vi "GetRobotPose.vi"() -> ()   [LabVIEW 2019]
uses:
  refnums.vi
  GRNF_GenericMotor.vi
  dsinstructions.vi
  sensors.vi
  dsdata.vi
  autoinfo.vi
panel:
  out "Y Position (in)":dbl=94.7
  out "X Position (in)":dbl=509.2
  out "Robot Position":cluster{dbl[], dbl[]}(graph)
  out "Heading (deg)":dbl format="%#_13g"
  in  "Plot Data":bool
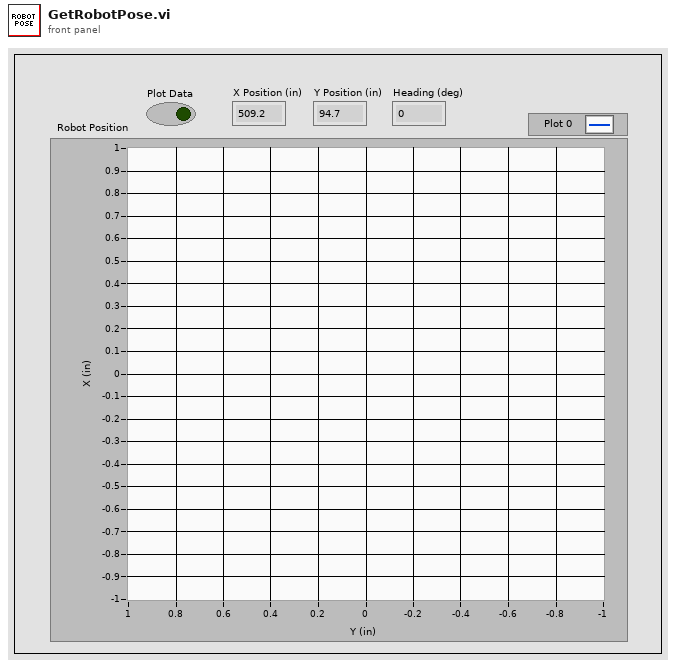
[diagram p1: front panel]
types:
  T1 = enum16{"Center", "North", "NorthWest", "West", "SouthWest", "South", "SouthEast", "East", "NorthEast"}
  T2 = typedef "WPI_MotorControlDeviceRef.ctl" = cluster{"DeviceStatus":errorcluster, "Type":T3, "PWM":cluster{"PWM Channel":T4, "DeadBand":T5}, "CAN":cluster{"Device Number":u8, "SetOutput VI Ref":variant, "GetOutput VI Ref":variant, "Enable VI Ref":variant, "Disable VI Ref":variant, "Data":variant}, "Invert":bool, "DIO PWM":cluster{"PWM \"Enable\" Channel":T4, "DIOChannel":T6, "PWM Rate":dbl}}
  T3 = typedef "WPI_MotorControlType.ctl" = enum16{"PWM", "CAN", "DIO PWM"}
  T4 = typedef "FPGA_DIOPWMChannel.ctl" = enum8{"PWM 0", "PWM 1", "PWM 2", "PWM 3", "PWM 4", "PWM 5", "PWM 6", "PWM 7", "PWM 8", "PWM 9", "PWM MXP 0", "PWM MXP 1", "PWM MXP 2", "PWM MXP 3", "PWM MXP 4", "PWM MXP 5", "PWM MXP 6", "PWM MXP 7", "PWM MXP 8", "PWM MXP 9", "Invalid"}
  T5 = typedef "WPI_PWMDeadband.ctl" = cluster{"Name":string, "maxPositivePwm":i32, "minPositivePwm":i32, "centerPwm":i32, "maxNegativePwm":i32, "minNegativePwm":i32, "angularRange":u16}
  T6 = typedef "FPGA_DIOChannel.ctl" = enum8{"DIO 0", "DIO 1", "DIO 2", "DIO 3", "DIO 4", "DIO 5", "DIO 6", "DIO 7", "DIO 8", "DIO 9", "DIO MXP 0", "DIO MXP 1", "DIO MXP 2", "DIO MXP 3", "DIO MXP 4", "DIO MXP 5", "DIO MXP 6", "DIO MXP 7", "DIO MXP 8", "DIO MXP 9", "DIO MXP 10", "DIO MXP 11", "DIO MXP 12", "DIO MXP 13", "DIO MXP 14", "DIO MXP 15", "SPI Port CS1", "SPI Port CS2", "SPI Port CS3", "SPI Port MISO", "SPI Port MOSI", "Invalid"}
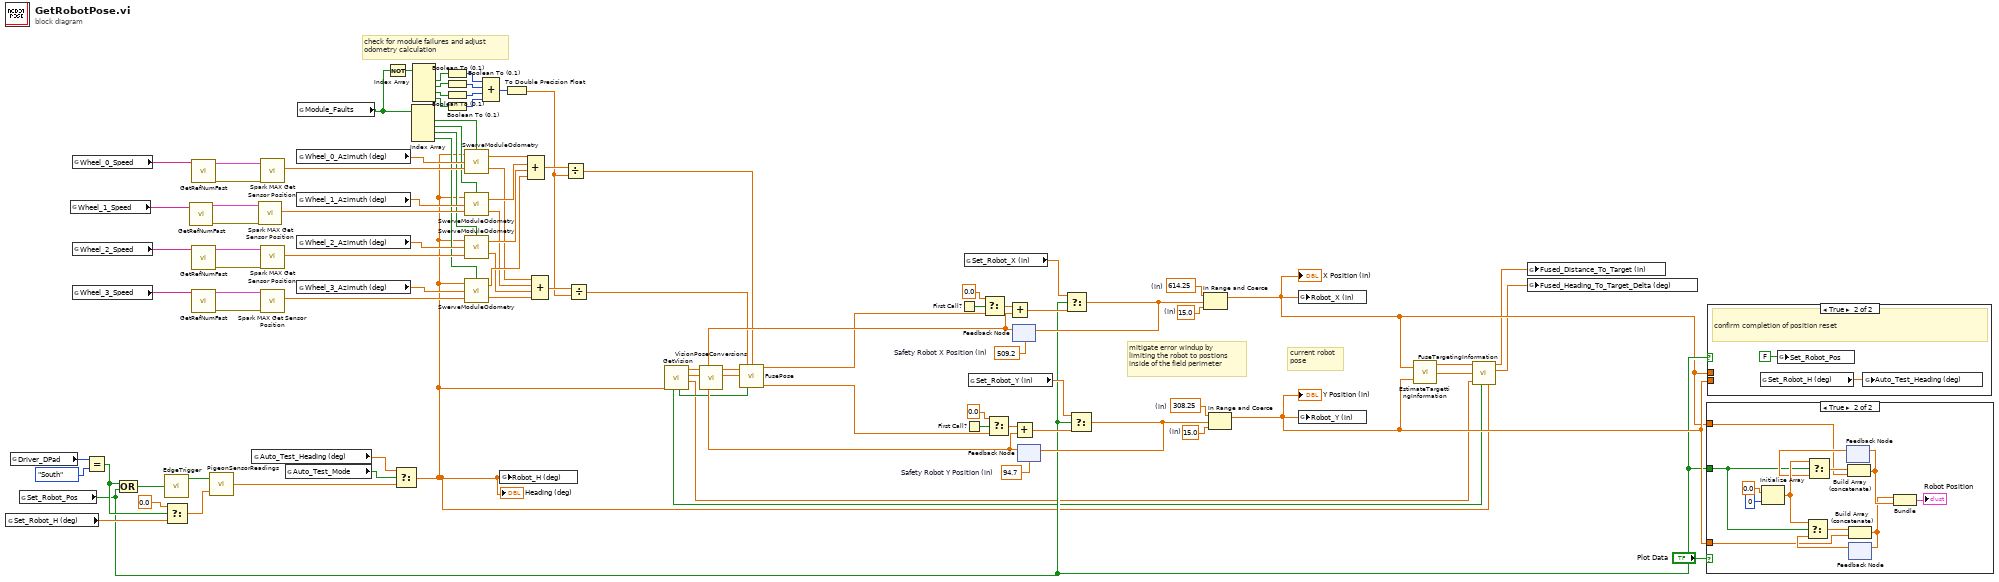
[diagram p0: block diagram]
diagram:
  w29 = 308.25  # (in)
  w30 = 15.0  # (in)
  w37 = 614.25  # (in)
  w38 = 15.0  # (in)
  w39 = 509.2  # Safety Robot X Position (in)
  w20 = 94.7  # Safety Robot Y Position (in)
  # "current robot\npose"
  # "mitigate error windup by\nlimiting the robot to postions\ninside of the field perimeter"
  # "check for module failures and adjust\nodometry calculation"
  n1 = global read "sensors.vi" "Set_Robot_H (deg)"() -> (w78:dbl)
  n2 = global read "dsinstructions.vi" "Driver_DPad"() -> (w54:T1)
  n3 = global read "sensors.vi" "Set_Robot_Pos"() -> (w12:bool)
  n4 = global read "refnums.vi" "Wheel_1_Speed"() -> (w46:string)
  n5 = global read "refnums.vi" "Wheel_0_Speed"() -> (w49:string)
  n6 = global read "refnums.vi" "Wheel_2_Speed"() -> (w43:string)
  n7 = global read "refnums.vi" "Wheel_3_Speed"() -> (w40:string)
  n8 = Equal?(x=w54, y=T1."South") -> (x = y?=w53:bool)
  n9 = Compound Arithmetic op=OR(w53, w12) -> (w77:bool)
  n10 = call "EdgeTrigger.vi"("Input Signal"=w77) -> ("Rising Edge Trigger"=w76:bool)  [unwired: 2 out]
  n11 = Select(t=0.0 ("f"), s=w53, f=w78) -> (s? t:f=w80:dbl)
  n12 = call-poly "GetRefNumFast.vi"("RefNum Name"=w46) -> ("Error"=w47:errorcluster, "Device Reference"=w48:T2)  [unwired: 5 in]
  n13 = call-poly "GetRefNumFast.vi"("RefNum Name"=w49) -> ("Error"=w50:errorcluster, "Device Reference"=w51:T2)  [unwired: 5 in]
  n14 = call-poly "GetRefNumFast.vi"("RefNum Name"=w43) -> ("Error"=w44:errorcluster, "Device Reference"=w45:T2)  [unwired: 5 in]
  n15 = call-poly "GetRefNumFast.vi"("RefNum Name"=w40) -> ("Error"=w41:errorcluster, "Device Reference"=w42:T2)  [unwired: 5 in]
  n16 = call "PigeonSensorReadings.vi"("Reset Yaw (deg)"=w80, "Reset Yaw"=w76) -> ("Yaw (deg)"=w57:dbl)
  n17 = global read "autoinfo.vi" "Auto_Test_Heading (deg)"() -> (w55:dbl)
  n18 = call <vilib>:"Spark MAX Get Sensor Position.vi"("error in (no error)"=w47, "MotorControlDevRef in"=w48) -> ("Sensor Position"=w94:dbl)  [unwired: 6 in, 3 out]
  n19 = call <vilib>:"Spark MAX Get Sensor Position.vi"("error in (no error)"=w50, "MotorControlDevRef in"=w51) -> ("Sensor Position"=w96:dbl)  [unwired: 6 in, 3 out]
  n20 = call <vilib>:"Spark MAX Get Sensor Position.vi"("error in (no error)"=w44, "MotorControlDevRef in"=w45) -> ("Sensor Position"=w93:dbl)  [unwired: 6 in, 3 out]
  n21 = call <vilib>:"Spark MAX Get Sensor Position.vi"("error in (no error)"=w41, "MotorControlDevRef in"=w42) -> ("Sensor Position"=w74:dbl)  [unwired: 6 in, 3 out]
  n22 = global read "dsdata.vi" "Auto_Test_Mode"() -> (w56:bool)
  n23 = global read "sensors.vi" "Wheel_0_Azimuth (deg)"() -> (w95:dbl)
  n24 = global read "sensors.vi" "Wheel_1_Azimuth (deg)"() -> (w92:dbl)
  n25 = global read "sensors.vi" "Wheel_2_Azimuth (deg)"() -> (w91:dbl)
  n26 = global read "sensors.vi" "Wheel_3_Azimuth (deg)"() -> (w75:dbl)
  n27 = global read "sensors.vi" "Module_Faults"() -> (w73:bool[])
  n28 = Not(x=w73) -> (.not. x?=w72:bool[])
  n29 = Select(t=w55, s=w56, f=w57) -> (s? t:f=w5:dbl)
  "Heading (deg)" <- w5
  n30 = Index Array(array=w73) -> (element #1=w61:bool, element #2=w60:bool, element #3=w59:bool, element #4=w58:bool)  [unwired: 4 in]
  n31 = Index Array(array=w72) -> (element #1=w71:bool, element #2=w70:bool, element #3=w69:bool, element #4=w68:bool)  [unwired: 4 in]
  n32 = Boolean To (0,1)(Boolean=w71) -> (0, 1=w67:i16)
  n33 = Boolean To (0,1)(Boolean=w70) -> (0, 1=w66:i16)
  n34 = Boolean To (0,1)(Boolean=w69) -> (0, 1=w65:i16)
  n35 = Boolean To (0,1)(Boolean=w68) -> (0, 1=w64:i16)
  n36 = call "SwerveModuleOdometry.vi"("Module Fault"=w61, "Wheel Distance (native)"=w96, "Wheel Azimuth (deg)"=w95, "Robot Heading(deg)"=w5) -> ("Delta Y (in)"=w81:dbl, "Delta X (in)"=w90:dbl)
  n37 = call "SwerveModuleOdometry.vi"("Module Fault"=w60, "Wheel Distance (native)"=w94, "Wheel Azimuth (deg)"=w92, "Robot Heading(deg)"=w5) -> ("Delta Y (in)"=w82:dbl, "Delta X (in)"=w89:dbl)
  n38 = call "SwerveModuleOdometry.vi"("Module Fault"=w59, "Wheel Distance (native)"=w93, "Wheel Azimuth (deg)"=w91, "Robot Heading(deg)"=w5) -> ("Delta Y (in)"=w83:dbl, "Delta X (in)"=w88:dbl)
  n39 = call "SwerveModuleOdometry.vi"("Module Fault"=w58, "Wheel Distance (native)"=w74, "Wheel Azimuth (deg)"=w75, "Robot Heading(deg)"=w5) -> ("Delta Y (in)"=w84:dbl, "Delta X (in)"=w87:dbl)
  n40 = Compound Arithmetic op=ADD(w67, w66, w65, w64) -> (w63:i16)
  n41 = global write "sensors.vi" "Robot_H (deg)"(w5) -> ()
  n42 = To Double Precision Float(number=w63) -> (double precision float=w62:dbl)
  n43 = Compound Arithmetic op=ADD(w90, w89, w88, w87) -> (w86:dbl)
  n44 = Compound Arithmetic op=ADD(w81, w82, w83, w84) -> (w85:dbl)
  n45 = Divide(x=w86, y=w62) -> (x/y=w14:dbl)
  n46 = Divide(x=w85, y=w62) -> (x/y=w13:dbl)
  n47 = call "GetVision.vi"("Robot_H (deg)"=w5) -> ("LimeLight Raw Horizontal Offset (deg)"=w6:dbl, "LimeLight Raw X (in)"=w18:dbl, "LimeLight Raw Z (in)"=w19:dbl, "LimeLight Pose Valid"=w8:bool, "LimeLight Valid"=w7:bool)  [unwired: 6 in]
  n48 = First Call?() -> (First Call?: T/F=w35:bool)
  n49 = First Call?() -> (First Call?: T/F=w27:bool)
  n50 = global read "sensors.vi" "Set_Robot_X (in)"() -> (w31:dbl)
  n51 = global read "sensors.vi" "Set_Robot_Y (in)"() -> (w23:dbl)
  n52 = feedback #1(w39) -> (w21:dbl)
  n53 = feedback #2(w20) -> (w22:dbl)
  n54 = call "VisionPoseConversions.vi"("Previous Y Estimate (in)"=w22, "Previous X Estimate (in)"=w21, "LimeLight Raw X (in)"=w18, "LimeLight Raw Z (in)"=w19) -> ("deltaY (in)"=w10:dbl, "deltaX (in)"=w11:dbl)  [unwired: 6 in]
  n55 = call "FusePose.vi"("LimeLight deltaX"=w11, "Odometry deltaY"=w13, "Odometry deltaX"=w14, "LimeLight deltaY"=w10, "LimeLight Pose Valid"=w8) -> ("Fused deltaX"=w17:dbl, "Fused deltaY"=w16:dbl)  [unwired: 9 in]
  n56 = Select(t=0.0, s=w35, f=w17) -> (s? t:f=w36:dbl)
  n57 = Select(t=0.0, s=w27, f=w16) -> (s? t:f=w28:dbl)
  n58 = Add(x=w36, y=w21) -> (x+y=w33:dbl)
  n59 = Add(x=w28, y=w22) -> (x+y=w25:dbl)
  n60 = Select(t=w31, s=w12, f=w33) -> (s? t:f=w32:dbl)
  n61 = feedback-in #1(w32) -> ()
  n62 = Select(t=w23, s=w12, f=w25) -> (s? t:f=w24:dbl)
  n63 = feedback-in #2(w24) -> ()
  n64 = In Range and Coerce(upper limit=w37, x=w32, lower limit=w38) -> (coerced(x)=w9:dbl)  [unwired: 1 out]
  "X Position (in)" <- w9
  n65 = In Range and Coerce(upper limit=w29, x=w24, lower limit=w30) -> (coerced(x)=w15:dbl)  [unwired: 1 out]
  "Y Position (in)" <- w15
  n66 = global write "sensors.vi" "Robot_X (in)"(w9) -> ()
  n67 = global write "sensors.vi" "Robot_Y (in)"(w15) -> ()
  n68 = call "EstimateTargettingInformation.vi"("Robot X (in)"=w9, "Robot Y (in)"=w15) -> ("Estimated Distance to Target (in)"=w3:dbl, "Estimated Heading to Target (deg)"=w4:dbl)  [unwired: 1 in]
  n69 = call "FuseTargetingInformation.vi"("Robot_H (deg)"=w5, "LimeLight Valid"=w7, "LimeLight Raw Horizontal Offset (deg)"=w6, "Estimated Heading to Target (deg)"=w4, "Estimated Distance to Target (in)"=w3) -> ("Fused Heading to Target Delta (deg)"=w1:dbl, "Fused Distance to Target (in)"=w2:dbl)  [unwired: 5 in]
  n70 = global write "sensors.vi" "Fused_Distance_To_Target (in)"(w2) -> ()
  n71 = global write "sensors.vi" "Fused_Heading_To_Target_Delta (deg)"(w1) -> ()
  n72 = case shown="True" "Plot Data" {
    tunnel: w12 -> [_ w98]
    tunnel: w9 -> [_ w101]
    tunnel: w15 -> [_ w100]
    frame False {
    }
    frame True {
      n73 = Initialize Array(0.0 ("element"), 0 ("dimension size")) -> (w110:dbl[])
      n74 = feedback #3() -> (w106:dbl[])  [unwired: 1 in]
      n75 = Select(t=w110, s=w98, f=w106) -> (s? t:f=w107:dbl[])
      n76 = Build Array (concatenate)(w107, w101) -> (w105:dbl[])
      n77 = feedback-in #3(w105) -> ()
      n78 = feedback #4() -> (w108:dbl[])  [unwired: 1 in]
      n79 = Select(t=w110, s=w98, f=w108) -> (s? t:f=w109:dbl[])
      n80 = Build Array (concatenate)(w109, w100) -> (w104:dbl[])
      n81 = feedback-in #4(w104) -> ()
      n82 = Bundle(w104, w105) -> (→"Robot Position":cluster{dbl[], dbl[]})  [unwired: 1 in]
    }
  }
  n83 = case shown="True" w12 {
    tunnel: w9 -> [_ _]
    tunnel: w15 -> [_ _]
    frame False {
    }
    frame True {
      # "confirm completion of position reset"
      n84 = global read "sensors.vi" "Set_Robot_H (deg)"() -> (w111:dbl)
      n85 = global write "sensors.vi" "Set_Robot_Pos"(FALSE ("Set_Robot_Pos")) -> ()
      n86 = global write "autoinfo.vi" "Auto_Test_Heading (deg)"(w111) -> ()
    }
  }
